vi "TrackColorM5.vi"() -> ()   [LabVIEW 2015]
uses:
  <vilib>/Utility/miscctls.llb/LVPoint32TypeDef.ctl
panel:
  out "error out":errorcluster
  in  "Coords":T1
  out "picture":picture
  out "Waveform Chart 2":sgl[](graph)
  out "Waveform Chart":sgl(graph)
  out "Image Out 2":T2(plugin-control)
  in  "base path":path
  out "Image Out":T2(plugin-control)
  out "Image":T2(plugin-control)
  in  "Stop":bool
  out "Progress Bar":i32(slide) max=25 scale=1.0..25.0
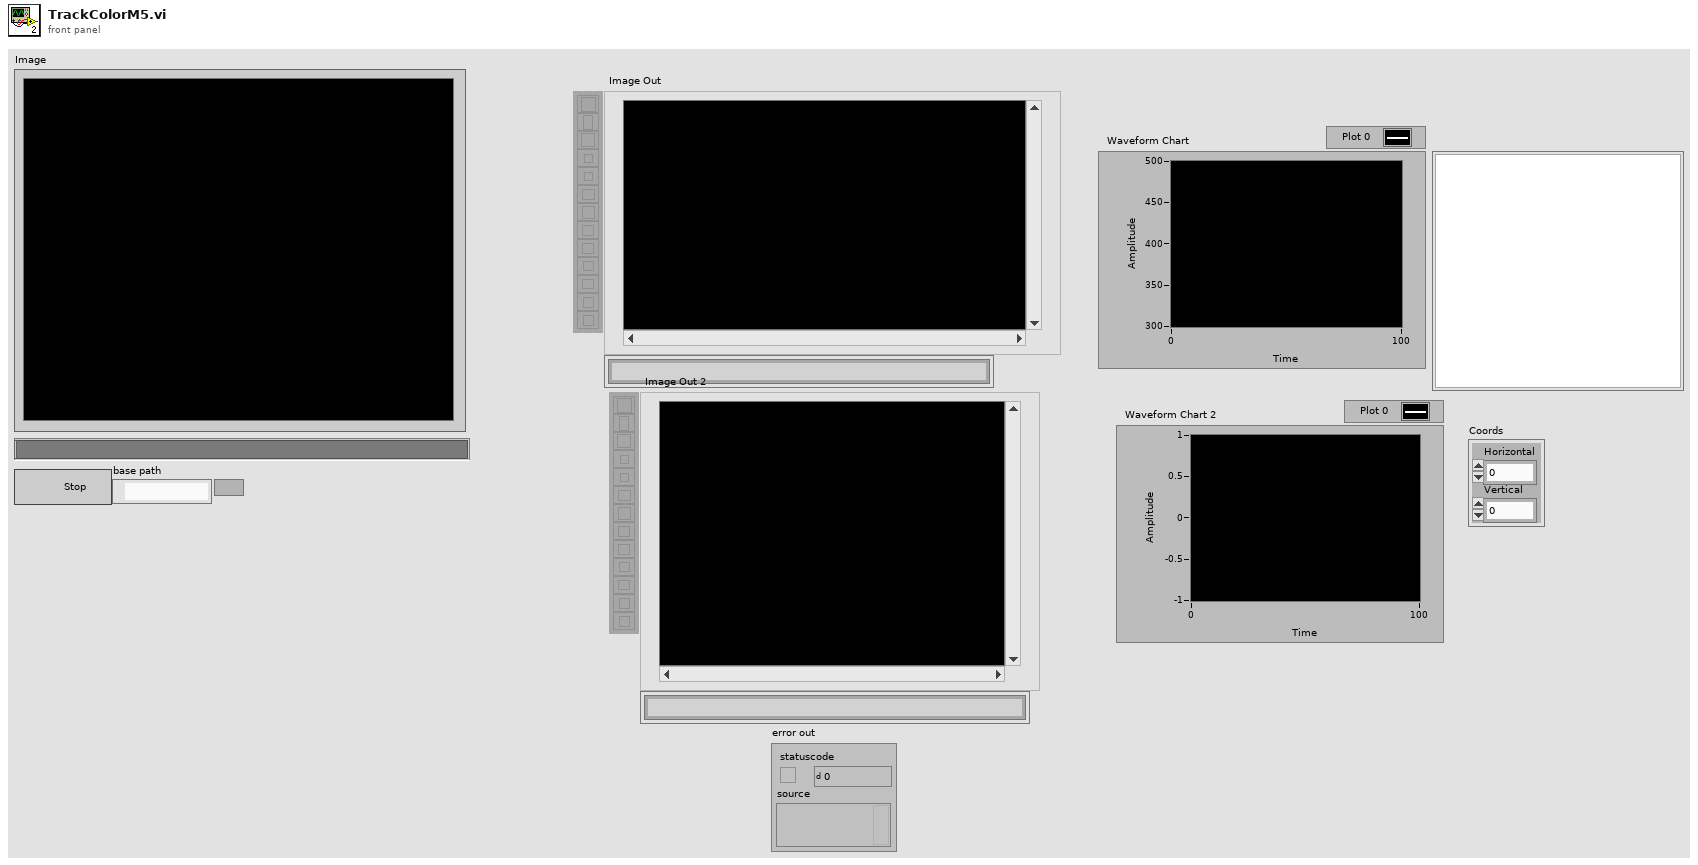
[diagram p1: front panel]
types:
  T1 = typedef "LVPoint32TypeDef.ctl" = cluster{"Horizontal":i32, "Vertical":i32}
  T2 = typedef "IMAQ Image.ctl" = refnum<image>
  T3 = typedef "IMAQ AVI2 Refnum.ctl" = refnum<k20>
  T4 = typedef "Image Type" = u32
  T5 = cluster{"Width":u32, "Height":u32, "Frames Per Second":u32, "Codec":string, "Has Data":bool}
  T6 = cluster{"Position":cluster{"x":sgl, "y":sgl}, "Angle":sgl, "Scale":sgl, "Score":sgl, "Bounding Box":cluster{"x":sgl, "y":sgl}[]}[]
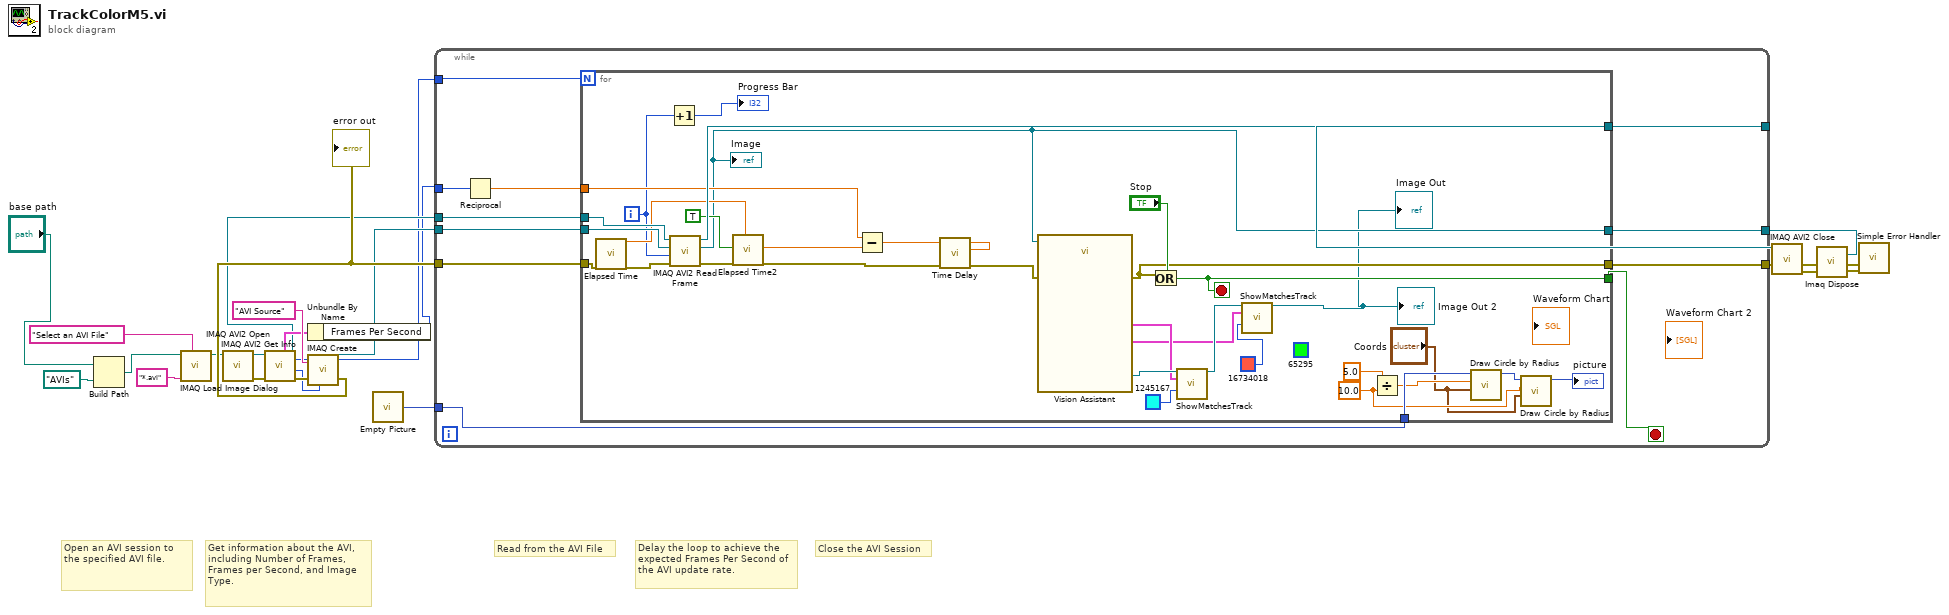
[diagram p0: block diagram]
diagram:
  # "Close the AVI Session"
  # "Read from the AVI File"
  # "Get information about the AVI, including Number of Frames, Frames per Second, and Image Type."
  # "Open an AVI session to the specified AVI file."
  # "Delay the loop to achieve the expected Frames Per Second of the AVI update rate."
  n1 = Build Path(base path="base path", name or relative path=path "AVIs") -> (appended path=w6:path)
  n2 = call "IMAQ Load Image Dialog"("Prompt"="Select an AVI File" ("prompt"), "Pattern"="*.avi", "Start Path"=w6) -> ("Path"=w5:path)  [unwired: 6 in, 2 out]
  n3 = call "IMAQ AVI2 Open"("AVI File Path"=w5) -> ("error out"=w20:errorcluster, "AVI Refnum"=w19:T3)  [unwired: 2 in, 7 out]
  n4 = call "IMAQ AVI2 Get Info"("error in (no error)"=w20, "AVI Refnum"=w19) -> ("error out"=w16:errorcluster, "Image Type"=w10:T4, "Number of Frames"=w3:u32, "AVI Refnum (duplicate)"=w13:T3, "Frame Data"=w21:T5)  [unwired: 5 out]
  n5 = Unbundle By Name(w21) -> ("Frames Per Second"=w9:u32)
  n6 = call "IMAQ Create"("Image Name"="AVI Source", "Image Type"=w10, "error in (no error)"=w16) -> ("New Image"=w14:T2, "error out"=w15:errorcluster)  [unwired: 1 in, 1 out]
  "error out" <- w15
  n7 = call "Empty Picture"() -> ("empty picture"=w1:picture)
  n8 = while {
    tunnel: [w34] -> w18
    tunnel: [w33] -> w17
    tunnel: w15 -> [w32]
    tunnel: w14 -> [w31]
    tunnel: w13 -> [w30]
    tunnel: [w29] -> w11
    tunnel: w9 -> [w28]
    tunnel: w3 -> [w26]
    tunnel: w1 -> [w24]
    stop <- w25 stop-if-true
    n9 = Reciprocal(x=w28) -> (1/x=w27:dbl)
    n10 = for {
      N: w26 -> [_]
      tunnel: w31 -> [w66]
      tunnel: [w65] -> w33
      tunnel: [w49] -> w34
      tunnel: w32 -> [w64]
      tunnel: w30 -> [w67]
      tunnel: [w52] -> w29
      tunnel: w27 -> [w62]
      tunnel: [w51] -> w25
      tunnel: w24 -> [w42]
      i -> [w54]
      stop <- w51 stop-if-true
      w38 = sgl 10.0 ("y")
      (unwired) u32 65295 ("Color")
      n11 = call "Elapsed Time"("error in (no error)"=w64) -> ("Present (s)"=w60:dbl, "error out"=w63:errorcluster)  [unwired: 11 in, 6 out]
      n12 = Increment(x=w54) -> (x+1=→"Progress Bar":i32)
      n13 = call "IMAQ AVI2 Read Frame"("error in (no error)"=w63, "Frame Number"=w54, "Image"=w66, "AVI Refnum"=w67) -> ("error out"=w58:errorcluster, "Image Out"=w52:T2, "AVI Refnum (duplicate)"=w65:T3)  [unwired: 5 out]
      "Image" <- w52
      n14 = call "Elapsed Time2"("Reset"=TRUE, "error in (no error)"=w58, "Set Start Time (s)"=w60) -> ("Elapsed Time (s)"=w57:dbl, "error out"=w56:errorcluster)  [unwired: 9 in, 6 out]
      n15 = Subtract(x=w62, y=w57) -> (x-y=w61:dbl)
      n16 = call "Time Delay"("error in (no error)"=w56, "Delay Time (s)"=w61) -> ("error out"=w50:errorcluster)  [unwired: 9 in]
      n17 = call "Vision Assistant"("Image In"=w52, "error in"=w50) -> ("Image Out"=w48:T2, "Matches (Color Location 1)"=w47:T6, "Matches (Color Location 2)"=w43:T6, "error out"=w49:errorcluster)  [unwired: 21 in, 1 out]
      n18 = Or(x=w49, y="Stop") -> (x .or. y?=w51:bool)
      n19 = call "ShowMatchesTrack.vi"("Refnum in"=w48, "Matches (Color Location 3)"=w47, "Color"=u32 1245167) -> ("Refnum out"=w46:T2)  [unwired: 7 in, 5 out]
      n20 = call "ShowMatchesTrack.vi"("Refnum in"=w46, "Matches (Color Location 3)"=w43, "Color"=u32 16734018) -> ("Refnum out"=→"Image Out" →"Image Out 2":T2)  [unwired: 7 in, 5 out]
      n21 = Divide(x=sgl 5.0, y=w38) -> (x/y=w41:sgl)
      n22 = call <vilib>:"Draw Circle by Radius.vi"("pixel center"="Coords", "radius"=w41, "picture"=w42) -> ("new picture"=w40:picture)  [unwired: 8 in]
      n23 = call <vilib>:"Draw Circle by Radius.vi"("pixel center"="Coords", "radius"=w38, "picture"=w40) -> ("new picture"=→"picture":picture)  [unwired: 8 in]
    }
  }
  n24 = call "IMAQ AVI2 Close"("error in (no error)"=w18, "AVI Refnum"=w17) -> ("error out"=w12:errorcluster)  [unwired: 9 out]
  n25 = call "Imaq Dispose"("Image"=w11, "error in (no error)"=w12) -> ("error out"=w22:errorcluster)  [unwired: 1 in, 3 out]
  n26 = call <vilib>:"Simple Error Handler.vi"("error in (no error)"=w22) -> ()  [unwired: 1 in, 8 out]
